vi "Build_from_Wizard.vi"(8 "error in (no error)":errorcluster, 9 "programmatic":bool, 10 "preview":bool, 11 "AB_Build in":refnum<class "AB_Build.lvclass">) -> (0 "error out":errorcluster, 1 "GeneratedFiles":path[](array[path]), 2 "Dependencies":T1[](array[typedef]), 3 "AB_Build out":refnum<class "AB_Build.lvclass">)   [LabVIEW 2020, in "AB_Build.lvclass"]
uses:
  <vilib>/AppBuilder/AB_Classes/Build/AB_Build.lvclass
  <vilib>/AppBuilder/AB_Dependency.ctl
  <vilib>/Utility/lvfile.llb/LVFileType.ctl
  <vilib>/AppBuilder/AB_Classes/Build/AB_Build.lvclass/AB_Build.ctl
  <resource>/Framework/Providers/Common/provcom_ProgressBar_Events.ctl
  <resource>/Framework/Providers/API/mxLvBuildError.ctl
  <resource>/Framework/Providers/Common/provcom_ProgressBar_Dialog_Text.ctl
  <resource>/Framework/Providers/Common/provcom_StringGlobals.vi
  <vilib>/Utility/lvfile.llb/NI_FileType.lvlib
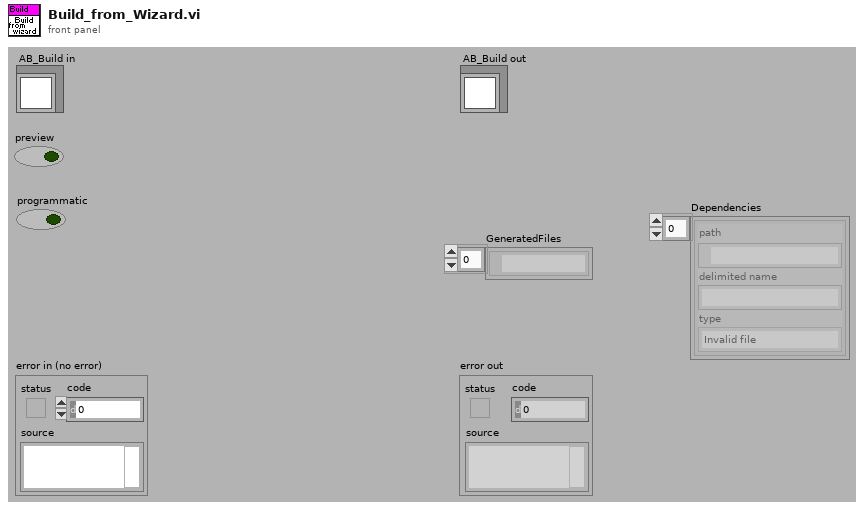
[diagram p1: front panel]
types:
  T1 = typedef "AB_Dependency.ctl" = cluster{"path":path, "delimited name":string, "type":T2}
  T2 = typedef "NI_FileType.lvlib/LVFileType.ctl" = enum32{"Invalid file", "Unknown type", "Instrument", "Control", "Polymorphic VI", "Project", "Library", "LVClass", "XControl", "XNode", "Shared library", ".NET assembly", "ActiveX interface", "CIN", "Run-time menu", "Palette menu", "Help file", "LLB", "XNode Edit Dependency", "Class Private Data Control", "Statechart", "MathScript .m file", "Ladder Diagram", "LVLibp", "XNode Build Dependency"}
  T3 = typedef "provcom_ProgressBar_Events.ctl" = cluster{"newJob":refnum<user-event>, "newItem":refnum<user-event>, "errorMsg":T4, "cancel":refnum<user-event>}
  T4 = typedef "mxLvBuildError.ctl" = refnum<user-event>
  T5 = typedef "provcom_ProgressBar_Dialog_Text.ctl" = cluster{"Operation action label":string, "Window title":string, "Expand text":string}
  T6 = typedef "ItemRef.ctl" = u64
  T7 = typedef "mxLvBuildNewJob.ctl" = refnum<user-event>
  T8 = typedef "mxLvBuildNewItem.ctl" = refnum<user-event>
  T9 = typedef "mxLvBuildCancel.ctl" = refnum<user-event>
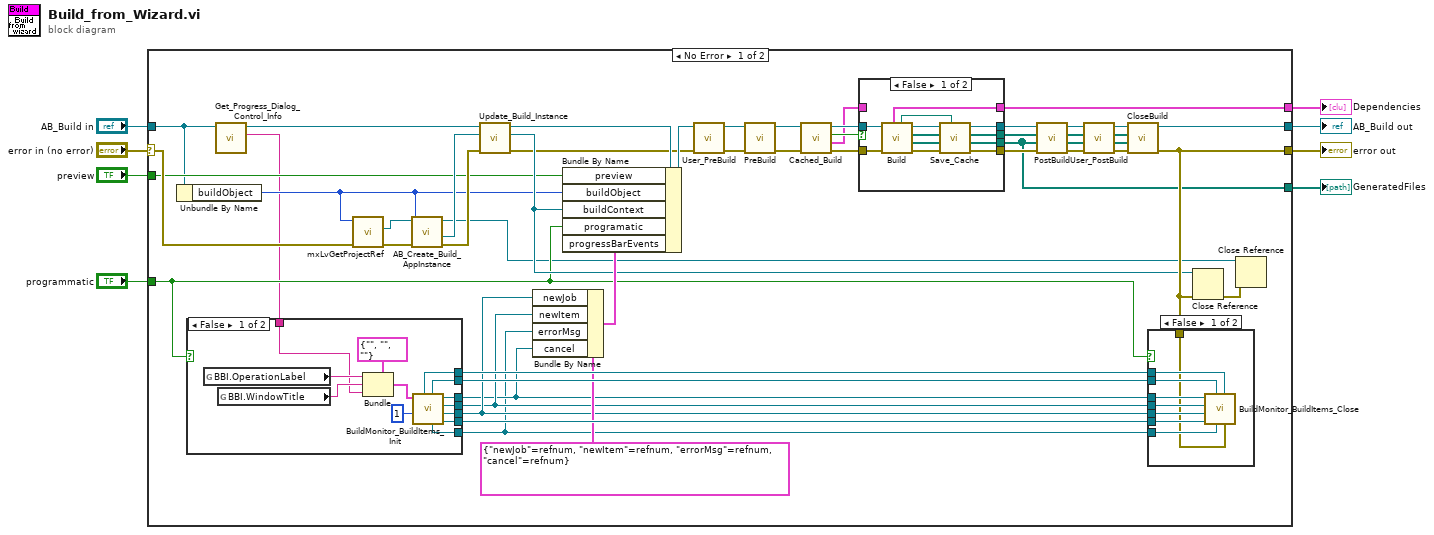
[diagram p0: block diagram]
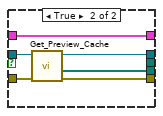
[diagram p2: hidden frame]
diagram:
  n1 = case shown="No Error" "error in (no error)" {
    selector: "error in (no error)" -> [w46 w98]
    tunnel: [w47 w98] -> w7
    tunnel: [w54 w97] -> w5
    tunnel: "AB_Build in" -> [w15 w97]
    tunnel: "preview" -> [w23 _]
    tunnel: "programmatic" -> [w17 _]
    tunnel: [w24 _] -> w2
    tunnel: [w9 _] -> w1
    frame No Error {
      n2 = Unbundle By Name(w15) -> ("buildObject"=w16:T6)
      n3 = call-dynamic "Get_Progress_Dialog_Control_Info.vi"("Build in"=w15) -> ("control text"=w13:string, "Build out"=w14:refnum<class "AB_Build.lvclass">)  [unwired: 8 in, 1 out]
      n4 = case shown="False" w17 {
        tunnel: [w96 _] -> w57
        tunnel: [w95 _] -> w56
        tunnel: [w94 _] -> w55
        tunnel: [w93 _] -> w50
        tunnel: [w92 _] -> w51
        tunnel: [w91 _] -> w52
        tunnel: [w90 _] -> w49
        tunnel: w13 -> [w84 _]
        frame False {
          n5 = global read "provcom_StringGlobals.vi" "BBI.OperationLabel"() -> (w86:string)
          n6 = global read "provcom_StringGlobals.vi" "BBI.WindowTitle"() -> (w87:string)
          n7 = Bundle(cluster=T5 {"Operation action label"="", "Window title"="", "Expand text"=""} ("progressBar_DialogText"), "Operation action label"=w86, "Window title"=w87, "Expand text"=w84) -> (w85:T5)
          n8 = call <resource>:"BuildMonitor_BuildItems_Init.vi"("NumOfJobs"=u16 1, "progressBar_DialogText"=w85) -> ("Complete"=w96:refnum<user-event>, "NewJob"=w91:T7, "NewItem"=w92:T8, "Cancel event"=w93:T9, "Error event"=w90:T4, "ErrorOpenEvent"=w95:refnum<user-event>, "ErrorCloseEvent"=w94:refnum<user-event>)  [unwired: 3 in]
        }
        frame True {
        }
      }
      n9 = call <resource>:"mxLvGetProjectRef.vi"("error in"=w46, "Item"=w16) -> ("error out"=w45:errorcluster, "Project Refnum"=w44:refnum<vi>)  [unwired: 8 out]
      n10 = call <resource>:"AB_Create_Build_AppInstance.vi"("error in (no error)"=w45, "Object"=w16, "Project Refnum"=w44) -> ("error out"=w40:errorcluster, "Build app instance"=w43:refnum<vi>, "dup Project Refnum"=w12:refnum<vi>)  [unwired: 6 out]
      n11 = call-dynamic "Update_Build_Instance.vi"("error in (no error)"=w40, "AppInstanceForBuild in"=w43, "Build in"=w14) -> ("error out"=w30:errorcluster, "AppInstanceForBuild out"=w42:refnum<vi>, "Build out"=w41:refnum<class "AB_Build.lvclass">)  [unwired: 6 out]
      n12 = Bundle By Name(cluster=T3 {"newJob"=refnum, "newItem"=refnum, "errorMsg"=refnum, "cancel"=refnum} ("progressBarEvents"), "newJob"=w52, "newItem"=w51, "errorMsg"=w49, "cancel"=w50) -> (w48:T3)
      n13 = Bundle By Name(cluster=w41, "preview"=w23, "buildObject"=w16, "buildContext"=w42, "programatic"=w17, "progressBarEvents"=w48) -> (w31:refnum<class "AB_Build.lvclass">)
      n14 = call-dynamic "User_PreBuild.vi"("error in (no error)"=w30, "Build in"=w31) -> ("error out"=w29:errorcluster, "Build out"=w28:refnum<class "AB_Build.lvclass">)  [unwired: 8 in]
      n15 = call-dynamic "PreBuild.vi"("error in (no error)"=w29, "Build in"=w28) -> ("error out"=w22:errorcluster, "Build out"=w21:refnum<class "AB_Build.lvclass">)  [unwired: 1 in, 7 out]
      n16 = call-dynamic "Cached_Build.vi"("error in (no error)"=w22, "AB_Build in"=w21) -> ("error out"=w20:errorcluster, "Dependencies"=w10:T1[], "valid?"=w18:bool, "AB_Build out"=w19:refnum<class "AB_Build.lvclass">)  [unwired: 5 in, 1 out]
      n17 = case shown="False" w18 {
        tunnel: w19 -> [w69 w74]
        tunnel: w20 -> [w68 w73]
        tunnel: [w66 w75] -> w27
        tunnel: [w65 w72] -> w26
        tunnel: [w61 _] -> w25
        tunnel: [w62 w71] -> w24
        tunnel: [w58 w70] -> w9
        tunnel: w10 -> [_ w70]
        frame False {
          n18 = call-dynamic "Build.vi"("error in (no error)"=w68, "Build in"=w69) -> ("error out"=w64:errorcluster, "GeneratedFiles"=w63:path[], "GeneratedDirectories"=w60:path[], "Build out"=w67:refnum<class "AB_Build.lvclass">, "OutputDirectory"=w59:path, "Dependencies"=w58:T1[])  [unwired: 1 in, 3 out]
          n19 = call <vilib>:"Save_Cache.vi"("OutputDirectory"=w59, "error in (no error)"=w64, "GeneratedFiles"=w63, "GeneratedDirectories"=w60, "AB_Build in"=w67) -> ("error out"=w65:errorcluster, "GeneratedFiles out"=w62:path[], "GeneratedDirectories out"=w61:path[], "AB_Build out"=w66:refnum<class "AB_Build.lvclass">)  [unwired: 3 in]
        }
        frame True {
          n20 = call <vilib>:"Get_Preview_Cache.vi"("error in (no error)"=w73, "AB_Build in"=w74) -> ("error out"=w72:errorcluster, "GeneratedFiles"=w71:path[], "AB_Build out"=w75:refnum<class "AB_Build.lvclass">)  [unwired: 6 in, 1 out]
        }
      }
      n21 = call-dynamic "PostBuild.vi"("error in (no error)"=w26, "GeneratedFiles in"=w24, "GeneratedDirectories in"=w25, "Build in"=w27) -> ("error out"=w39:errorcluster, "GeneratedFiles out"=w32:path[], "GeneratedDirectories out"=w33:path[], "Build out"=w34:refnum<class "AB_Build.lvclass">)  [unwired: 4 out]
      n22 = call-dynamic "User_PostBuild.vi"("error in (no error)"=w39, "GeneratedFiles in"=w32, "GeneratedDirectories in"=w33, "Build in"=w34) -> ("error out"=w38:errorcluster, "GeneratedFiles out"=w37:path[], "GeneratedDirectories out"=w36:path[], "Build out"=w35:refnum<class "AB_Build.lvclass">)  [unwired: 4 in]
      n23 = call-dynamic "CloseBuild.vi"("error in (no error)"=w38, "GeneratedFiles"=w37, "GeneratedDirectories"=w36, "Build in"=w35) -> ("error out"=w47:errorcluster, "Build out"=w54:refnum<class "AB_Build.lvclass">)  [unwired: 6 out]
      n24 = case shown="False" w17 {
        tunnel: w57 -> [w83 _]
        tunnel: w56 -> [w82 _]
        tunnel: w55 -> [w81 _]
        tunnel: w50 -> [w80 _]
        tunnel: w51 -> [w79 _]
        tunnel: w52 -> [w78 _]
        tunnel: w49 -> [w77 _]
        tunnel: w47 -> [w76 _]
        frame False {
          n25 = call <resource>:"BuildMonitor_BuildItems_Close.vi"("error IO"=w76, "ErrorCloseEvent"=w81, "Error event"=w77, "ErrorOpenEvent"=w82, "Complete"=w83, "NewJob"=w78, "NewItem"=w79, "Cancel event"=w80) -> ()  [unwired: 1 in, 3 out]
        }
        frame True {
        }
      }
      n26 = Close Reference(reference=w42, error in (no error)=w47) -> (error out=w11:errorcluster)
      n27 = Close Reference(reference=w12, error in (no error)=w11) -> ()  [unwired: 1 out]
    }
    frame Error {
    }
  }
  "error out" <- w7
  "AB_Build out" <- w5
  "GeneratedFiles" <- w2
  "Dependencies" <- w1
